vi "FrameRateCalcs.vi"() -> ()   [LabVIEW 2022 SP3]
panel:
  out "Max # Tx  in SuperFrame":dbl
  out "Wavelengths One way Start":i32
  out "Wavelengths One way End":i32
  out "Sustatin Throughput?":bool
  out "Max PRF fro RT (kHz)":dbl
  out "nearest x128 Rcv Structure":i32
  out "Wavelengths in Window":i32
  out "effective Doppler PRF needed to resolve max flow (Hz)":dbl
  out "Single RT transmit time (us)":dbl
  out "PRF time (us)":dbl
  out "duration of one SuperFrame (s)":dbl
  out "Max # Compound images in one SuperFrame":dbl
  out "Samples/CH/sec":dbl
  out "Max effective image rate (Hz)":dbl
  in  "Cluster":T1={"Absolute Tx PRF (Hz)"=10.0, "Tx angles"=9.0, " extra time between ensemble bursts (ms)"=0.0, "Sound speed (mm/us)"=1.5, "end depth (mm)"=30.0, "Fc probe (MHz)"=20.0, "max flow mm/s"=25.0, "Samps/wavelength"=4, "F Tx"=20.0, "start depth (mm)"=30.0}
  out "Total ensemble duration (ms)":dbl
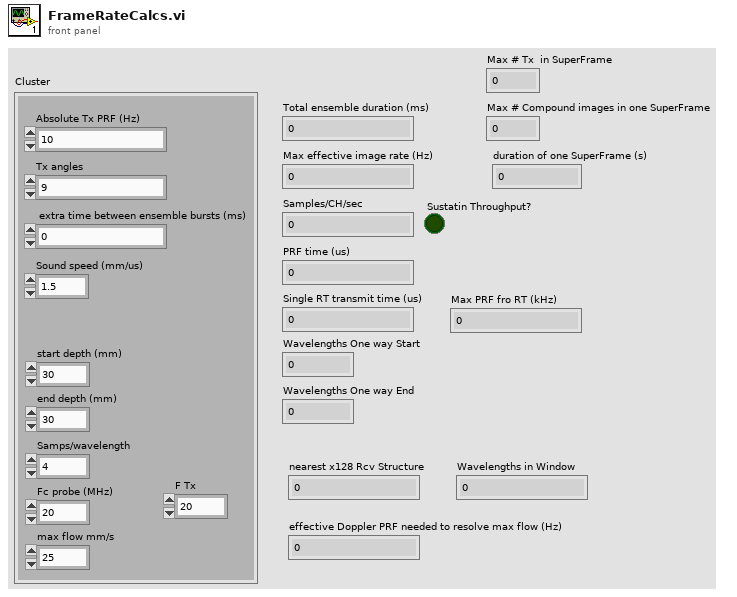
[diagram p1: front panel]
types:
  T1 = cluster{"Absolute Tx PRF (Hz)":dbl, "Tx angles":dbl, " extra time between ensemble bursts (ms)":dbl, "Sound speed (mm/us)":dbl, "end depth (mm)":dbl, "Fc probe (MHz)":dbl, "max flow mm/s":dbl, "Samps/wavelength":i8, "F Tx":dbl, "start depth (mm)":dbl}
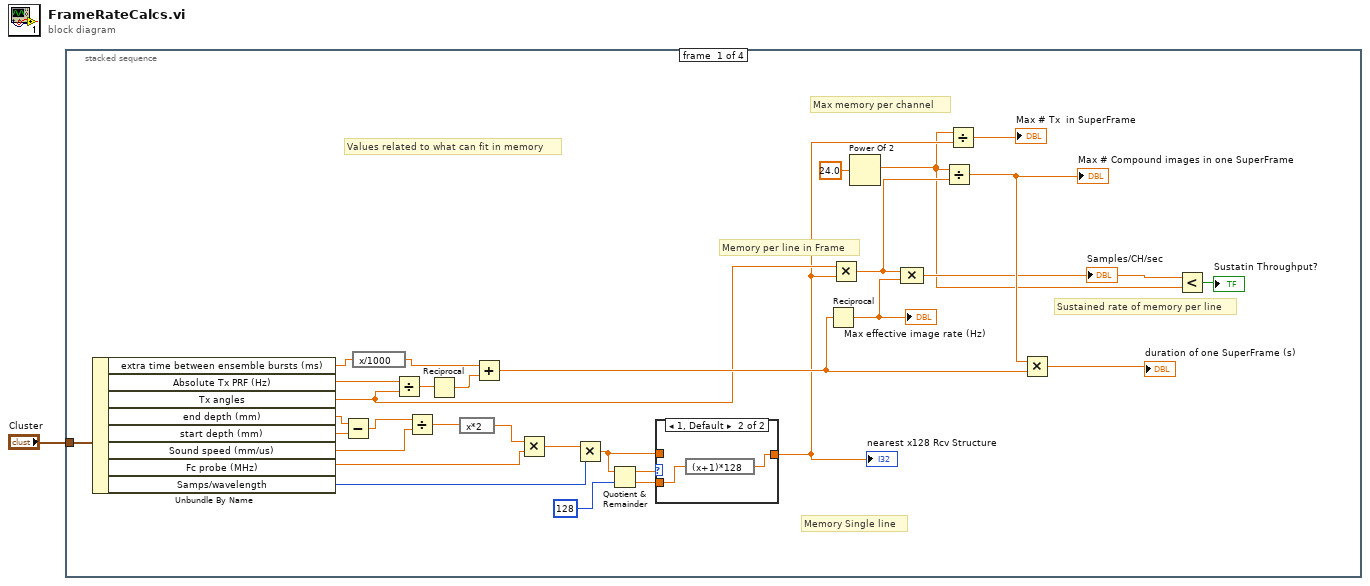
[diagram p0: block diagram]
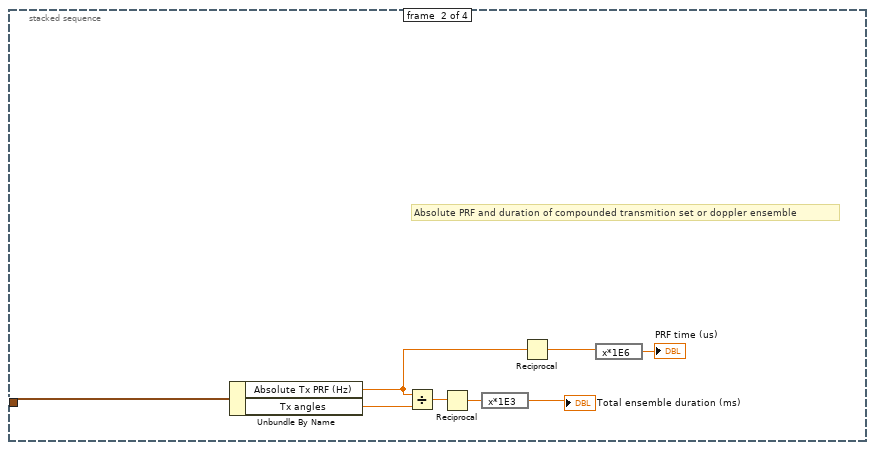
[diagram p3: hidden frame]
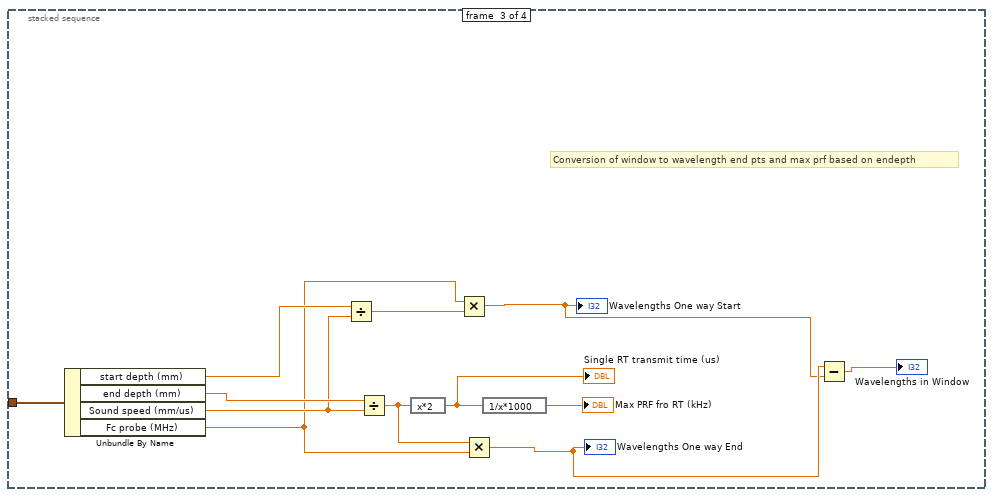
[diagram p4: hidden frame]
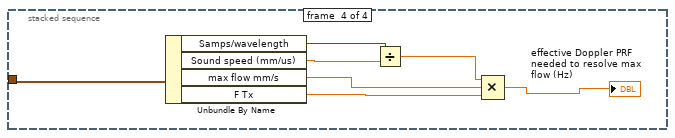
[diagram p5: hidden frame]
diagram:
  n1 = stacked-sequence {
    tunnel: "Cluster" -> [w32 w43 w55 w62]
    frame #0 {
      # "Sustained rate of memory per line"
      # "Memory per line in Frame"
      # "Memory Single line"
      # "Values related to what can fit in memory"
      # "Max memory per channel"
      n2 = Unbundle By Name(w32) -> ("extra time between ensemble bursts (ms)"=w6:dbl, "Absolute Tx PRF (Hz)"=w26:dbl, "Tx angles"=w10:dbl, "end depth (mm)"=w13:dbl, "start depth (mm)"=w14:dbl, "Sound speed (mm/us)"=w15:dbl, "Fc probe (MHz)"=w25:dbl, "Samps/wavelength"=w16:i8)
      n3 = Subtract(x=w13, y=w14) -> (x-y=w12:dbl)
      n4 = expression code="x/1000"(w6) -> (w5:dbl)
      n5 = Divide(x=w26, y=w10) -> (x/y=w31:dbl)
      n6 = Divide(x=w12, y=w15) -> (x/y=w24:dbl)
      n7 = Reciprocal(x=w31) -> (1/x=w28:dbl)
      n8 = expression code="x*2"(w24) -> (w19:dbl)
      n9 = Add(x=w5, y=w28) -> (x+y=w27:dbl)
      n10 = Multiply(x=w19, y=w25) -> (x*y=w18:dbl)
      n11 = Multiply(x=w18, y=w16) -> (x*y=w22:dbl)
      n12 = Quotient & Remainder(x=w22, y=128) -> (x-y*floor(x/y)=w21:dbl, floor(x/y)=w20:dbl)
      n13 = case shown="1, Default" w21 {
        tunnel: [w33 w35] -> w4
        tunnel: w22 -> [w33 _]
        tunnel: w20 -> [_ w34]
        frame 0 {
        }
        frame 1, Default {
          n14 = expression code="(x+1)*128"(w34) -> (w35:dbl)
        }
      }
      "nearest x128 Rcv Structure" <- w4
      n15 = Reciprocal(x=w27) -> (1/x=w30:dbl)
      "Max effective image rate (Hz)" <- w30
      n16 = Multiply(x=w10, y=w4) -> (x*y=w7:dbl)
      n17 = Power Of 2(x=24.0) -> (2^x=w2:dbl)
      n18 = Compound Arithmetic op=MULTIPLY(w7, w30) -> (w8:dbl)
      "Samples/CH/sec" <- w8
      n19 = Divide(x=w2, y=w7) -> (x/y=w9:dbl)
      "Max # Compound images in one SuperFrame" <- w9
      n20 = Divide(x=w2, y=w4) -> (x/y=→"Max # Tx  in SuperFrame":dbl)
      n21 = Multiply(x=w9, y=w27) -> (x*y=→"duration of one SuperFrame (s)":dbl)
      n22 = Less?(x=w8, y=w2) -> (x < y?=→"Sustatin Throughput?":bool)
    }
    frame #1 {
      # "Absolute PRF and duration of compounded transmition set or doppler ensemble"
      n23 = Unbundle By Name(w43) -> ("Absolute Tx PRF (Hz)"=w39:dbl, "Tx angles"=w41:dbl)
      n24 = Divide(x=w39, y=w41) -> (x/y=w42:dbl)
      n25 = Reciprocal(x=w42) -> (1/x=w37:dbl)
      n26 = expression code="x*1E3"(w37) -> (→"Total ensemble duration (ms)":dbl)
      n27 = Reciprocal(x=w39) -> (1/x=w40:dbl)
      n28 = expression code="x*1E6"(w40) -> (→"PRF time (us)":dbl)
    }
    frame #2 {
      # "Conversion of window to wavelength end pts and max prf based on endepth"
      n29 = Unbundle By Name(w55) -> ("start depth (mm)"=w51:dbl, "end depth (mm)"=w54:dbl, "Sound speed (mm/us)"=w50:dbl, "Fc probe (MHz)"=w49:dbl)
      n30 = Divide(x=w51, y=w50) -> (x/y=w47:dbl)
      n31 = Divide(x=w54, y=w50) -> (x/y=w46:dbl)
      n32 = expression code="x*2"(w46) -> (w53:dbl)
      "Single RT transmit time (us)" <- w53
      n33 = Multiply(x=w49, y=w47) -> (x*y=w44:dbl)
      "Wavelengths One way Start" <- w44
      n34 = Multiply(x=w46, y=w49) -> (x*y=w45:dbl)
      "Wavelengths One way End" <- w45
      n35 = expression code="1/x*1000"(w53) -> (→"Max PRF fro RT (kHz)":dbl)
      n36 = Subtract(x=w45, y=w44) -> (x-y=→"Wavelengths in Window":dbl)
    }
    frame #3 {
      n37 = Unbundle By Name(w62) -> ("Samps/wavelength"=w57:i8, "Sound speed (mm/us)"=w60:dbl, "max flow mm/s"=w59:dbl, "F Tx"=w58:dbl)
      n38 = Divide(x=w57, y=w60) -> (x/y=w61:dbl)
      n39 = Compound Arithmetic op=MULTIPLY(w61, w59, w58) -> (→"effective Doppler PRF needed to resolve max flow (Hz)":dbl)
    }
  }
